vi "process.vi"(8 "error in (no error)":errorcluster, 9 "Calling VI Reference i":refnum<vi>, 10 "GObj Refnum":refnum<vi>, 11 "DiagramObject in":refnum<class "GObject.lvclass">) -> (0 "error out":errorcluster, 3 "DiagramObject out":refnum<class "GObject.lvclass">)   [LabVIEW 2016, in "GObject.lvclass"]
uses:
  GObject.lvclass
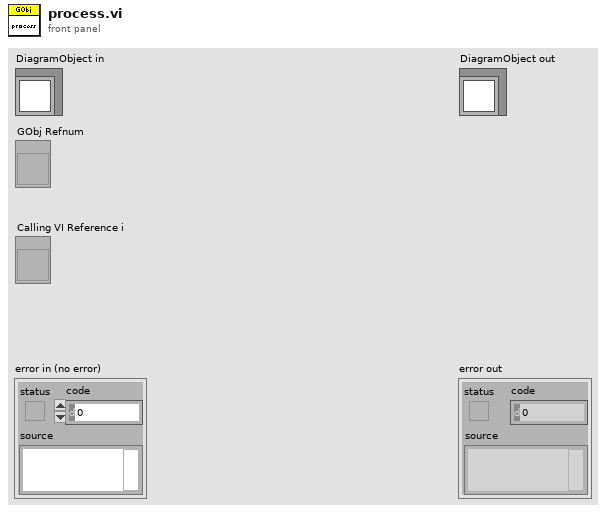
[diagram p1: front panel]
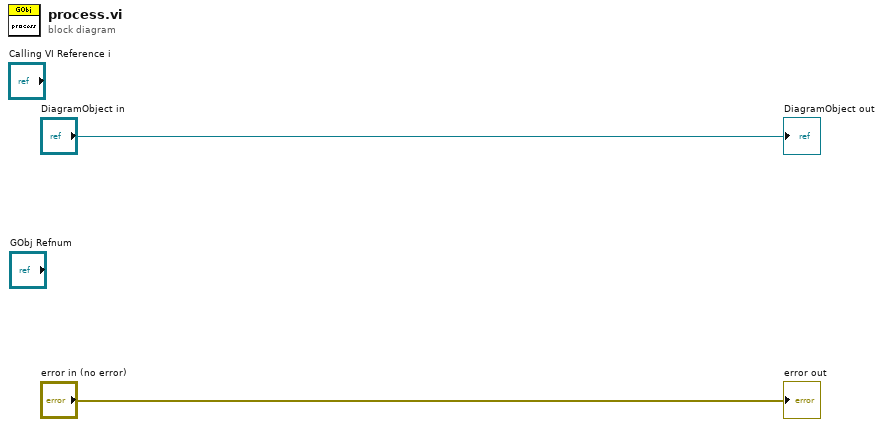
[diagram p0: block diagram]
diagram:
  "error out" <- "error in (no error)"
  "DiagramObject out" <- "DiagramObject in"
